vi "ExistingFile.vi"(8 "error in":errorcluster, 10 "Filename":string="Test") -> (0 "error out":errorcluster, 2 "file or folder exists?":bool)   [LabVIEW 2016]
uses:
  controls/Enum.ctl
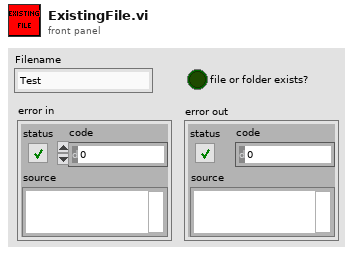
[diagram p1: front panel]
types:
  T1 = typedef "Enum.ctl" = enum16{"Init", "Read", "Write"}
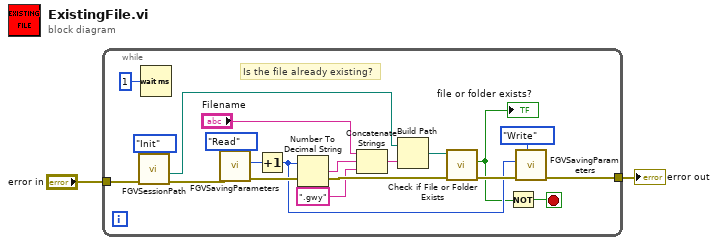
[diagram p0: block diagram]
diagram:
  n1 = while {
    tunnel: [w5] -> w2
    tunnel: "error in" -> [w3]
    stop <- w8 stop-if-true
    (unwired) Enum."Read" ("Enum")
    # "Is the file already existing?"
    n2 = call "FGVSessionPath.vi"("Enum"=Enum."Init", "error in"=w3) -> ("error out"=w4:errorcluster, "sessionPathOut"=w16:path)  [unwired: 8 in]
    n3 = Wait (ms)(milliseconds to wait=u32 1) -> ()  [unwired: 1 out]
    n4 = call "FGVSavingParameters.vi"("error in"=w4) -> ("error out"=w20:errorcluster, "#PicturesSavedOut"=w18:u32)  [unwired: 7 in, 2 out]
    n5 = Increment(x=w18) -> (x+1=w12:u32)
    n6 = Number To Decimal String(number=w12) -> (decimal integer string=w10:string)  [unwired: 1 in]
    n7 = Concatenate Strings("Filename", w10, ".gwy" ("string")) -> (w15:string)
    n8 = Build Path(base path=w16, name or relative path=w15) -> (appended path=w13:path)
    n9 = call <vilib>:"Check if File or Folder Exists.vi"("error in (no error)"=w20, "path"=w13) -> ("error out"=w19:errorcluster, "file or folder exists?"=w7:bool)  [unwired: 7 in, 1 out]
    "file or folder exists?" <- w7
    n10 = Not(x=w7) -> (.not. x?=w8:bool)
    n11 = call "FGVSavingParameters.vi"("Enum"=Enum."Write", "error in"=w19, "#PicturesSavedIn"=w12) -> ("error out"=w5:errorcluster)  [unwired: 5 in, 3 out]
  }
  "error out" <- w2
